vi "obstacle1.vi"(9 "Boolean":bool, 10 "f":i32, 11 "Position in":T1) -> (0 "deliver":bool, 3 "Position out":T1)   [LabVIEW 2014]
uses:
  <vilib>/Utility/miscctls.llb/LVPositionTypeDef.ctl
panel:
  out "skill":bool
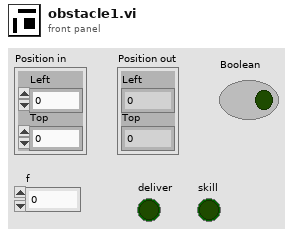
[diagram p1: front panel]
types:
  T1 = typedef "LVPositionTypeDef.ctl" = cluster{"Left":i32, "Top":i32}
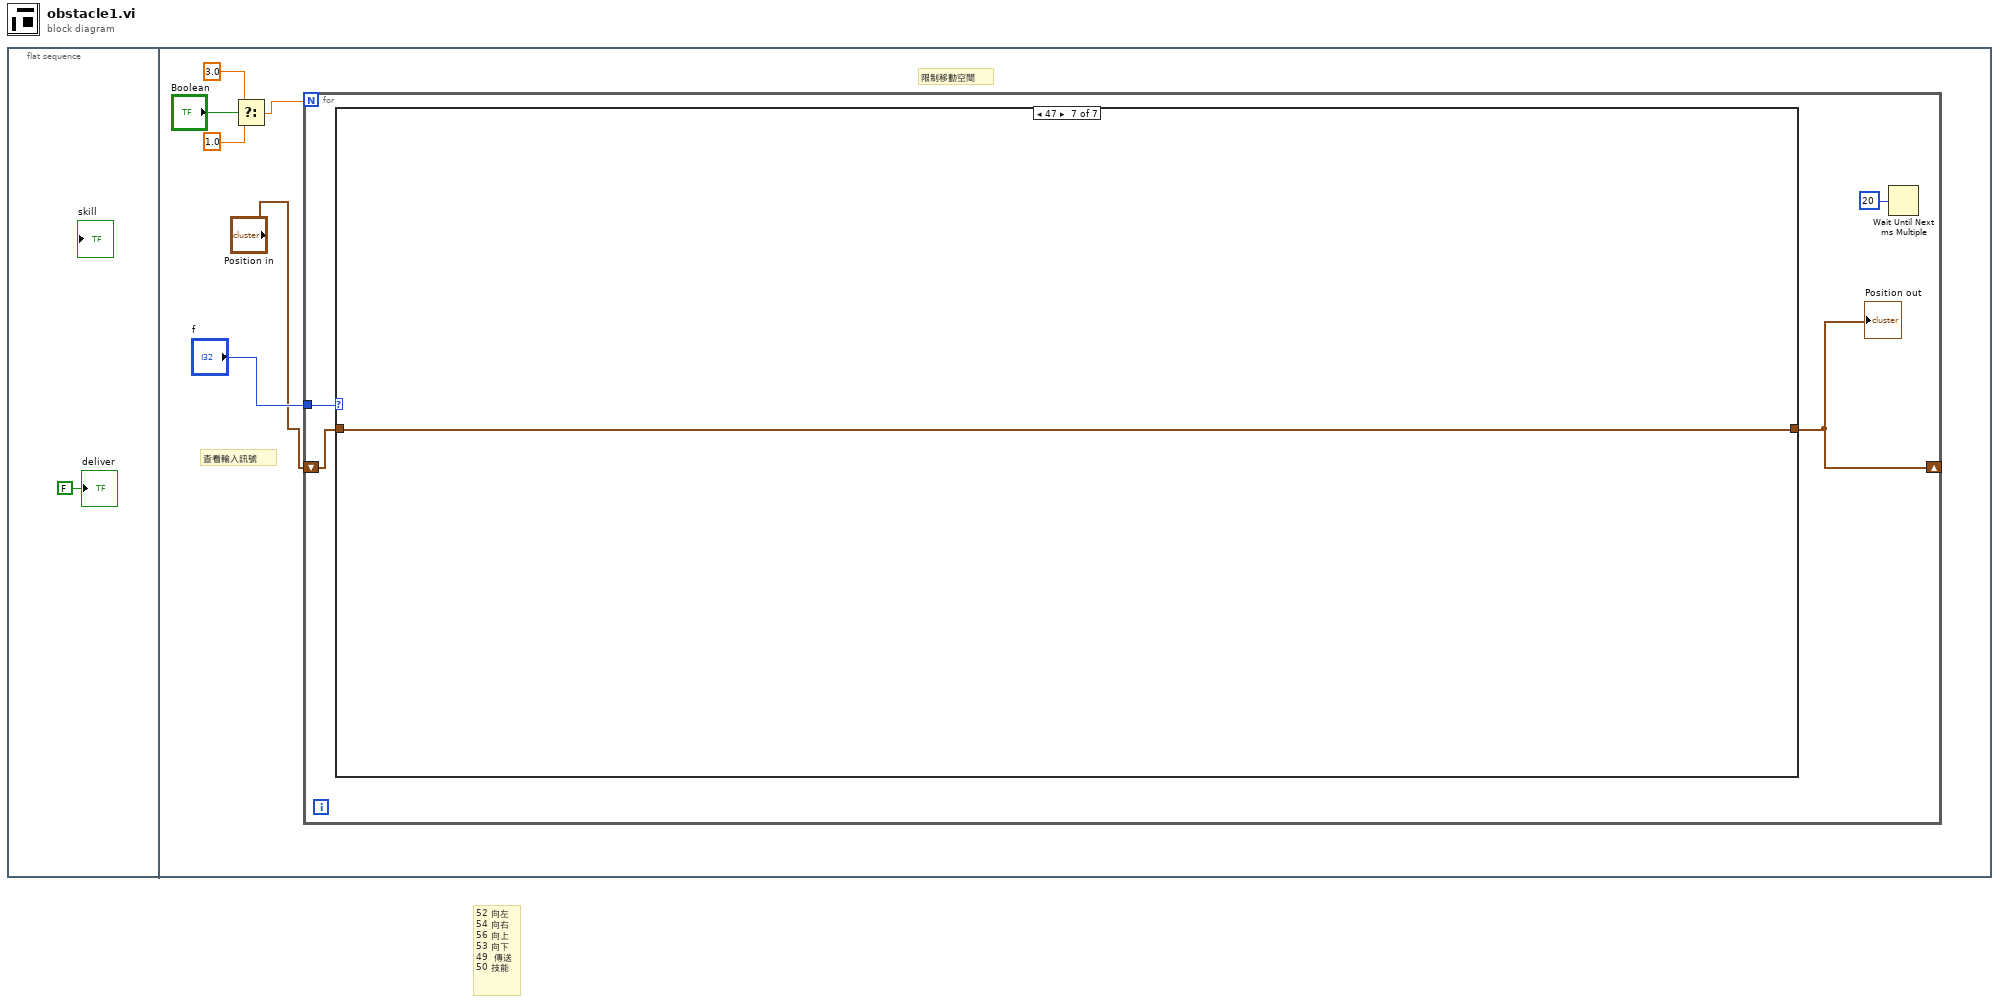
[diagram p0: block diagram]
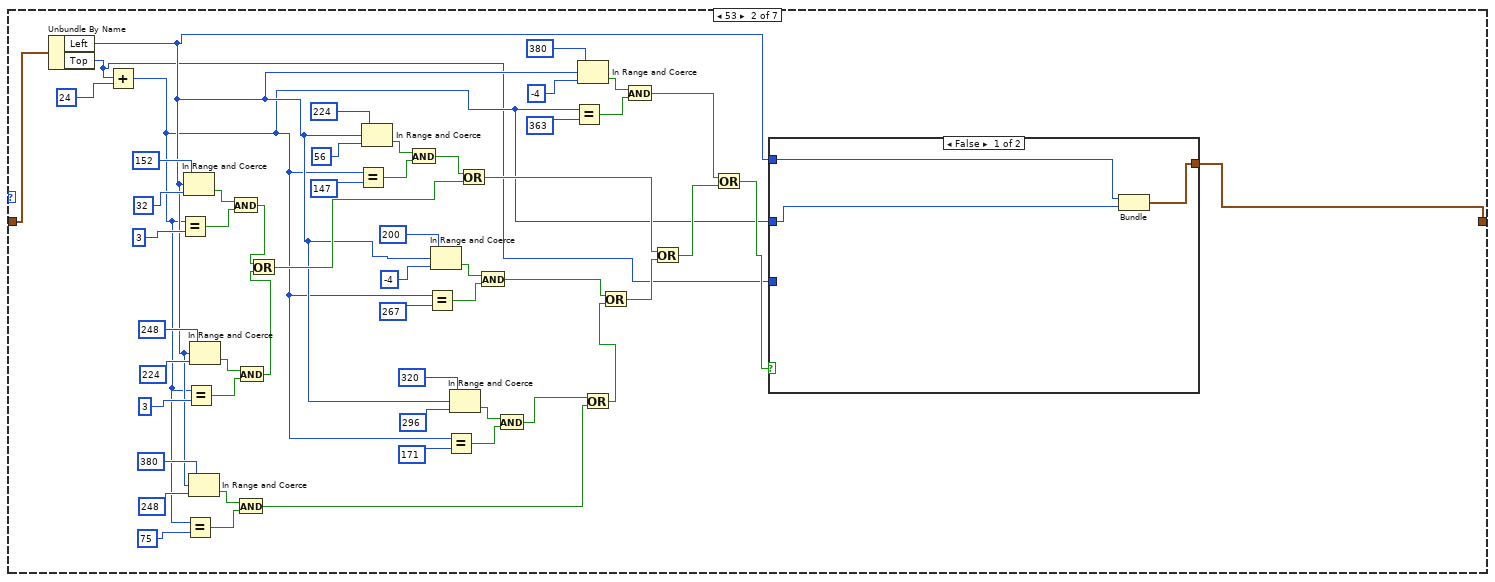
[diagram p3: hidden frame]
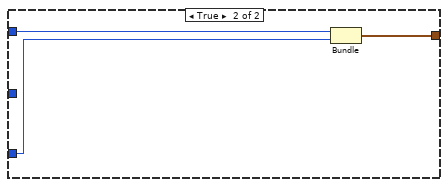
[diagram p4: hidden frame]
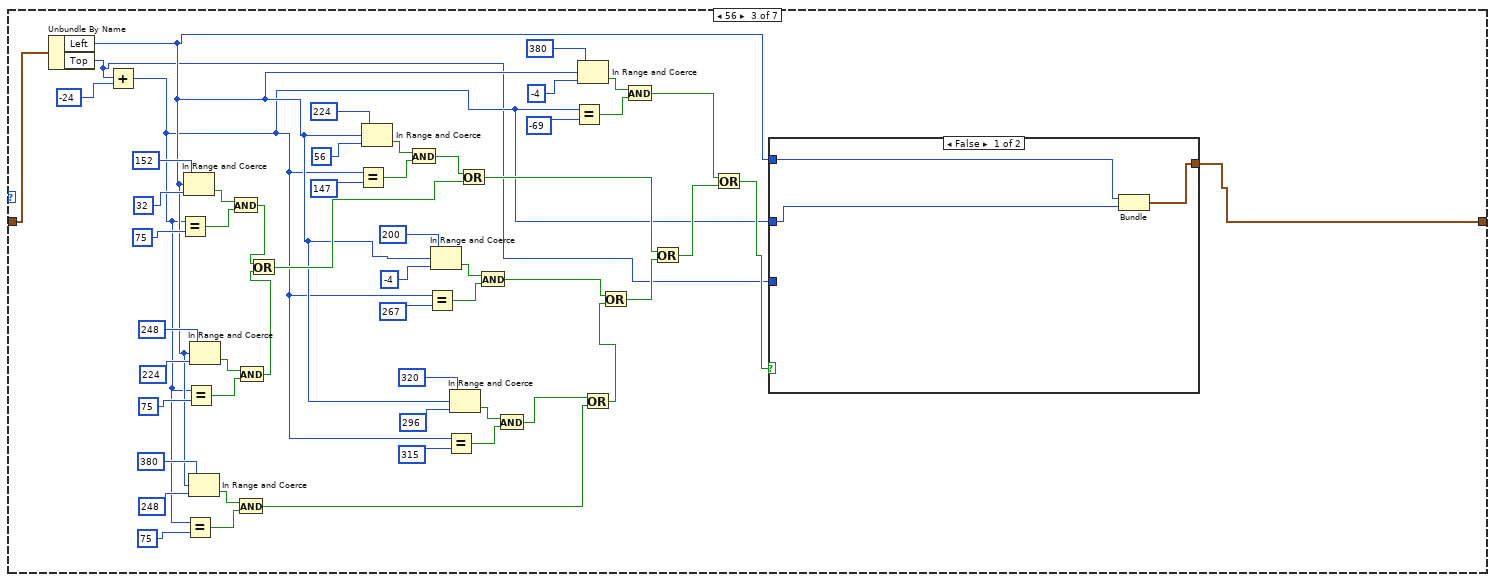
[diagram p5: hidden frame]
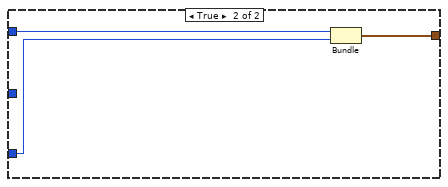
[diagram p6: hidden frame]
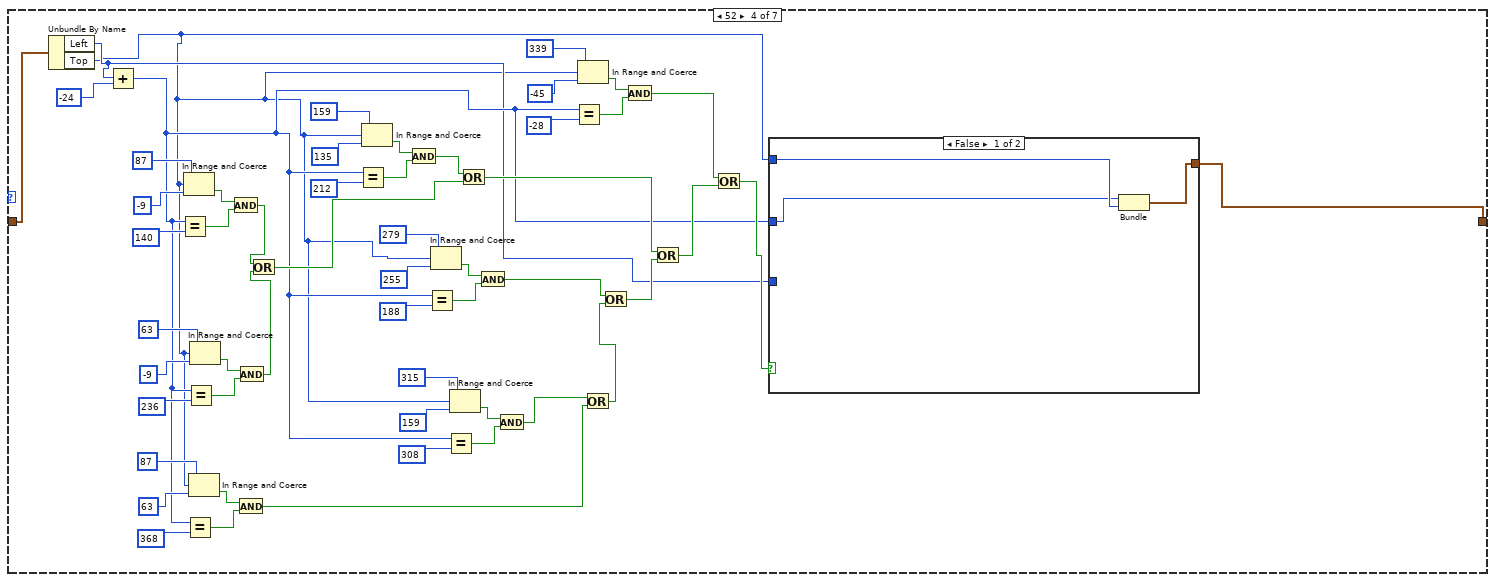
[diagram p7: hidden frame]
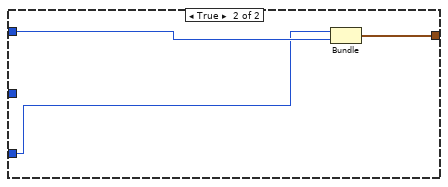
[diagram p8: hidden frame]
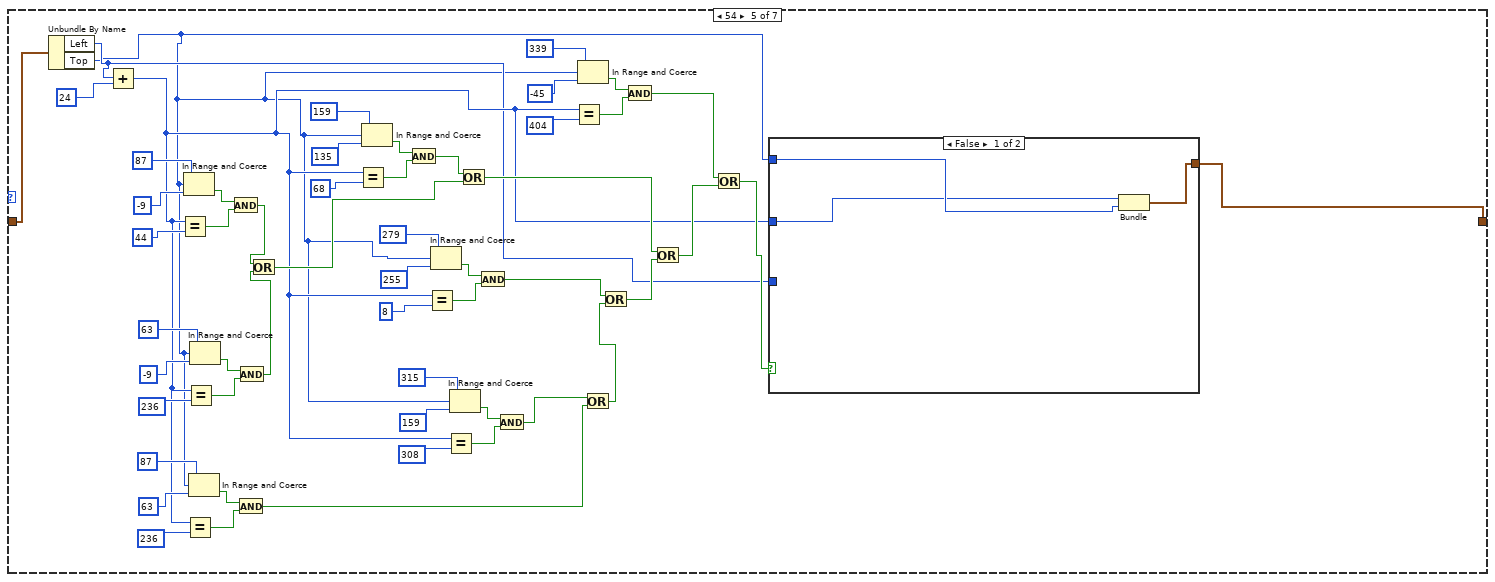
[diagram p9: hidden frame]
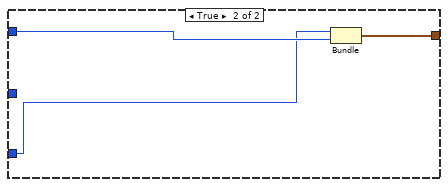
[diagram p10: hidden frame]
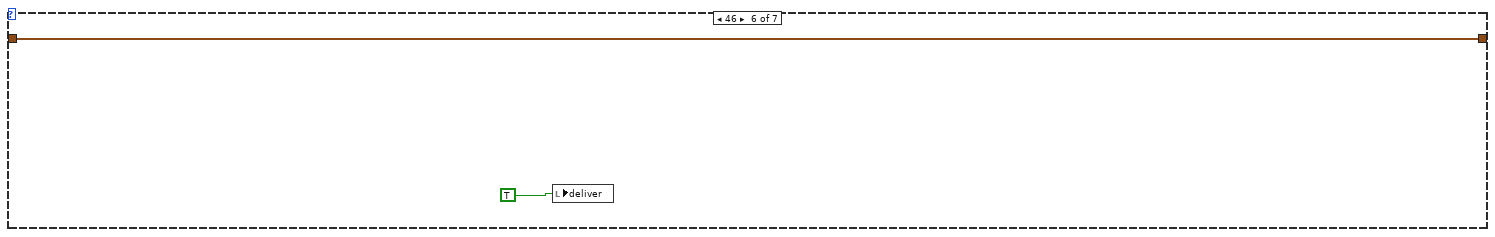
[diagram p11: hidden frame]
diagram:
  # "52 向左\n54 向右\n56 向上\n53 向下\n49  傳送\n50 技能"
  n1 = flat-sequence {
    frame #0 {
      "deliver" <- FALSE ("skill")
    }
    frame #1 {
      # "限制移動空間"
      # "查看輸入訊號"
      n2 = Select(t=3.0, s="Boolean", f=1.0) -> (s? t:f=w3:dbl)
      n3 = for {
        N: w3 -> [_]
        tunnel: "f" -> [w11]
        shift-right: [w10] -> _
        shift-left: "Position in" -> [w9]
        n4 = case shown="47" w11 {
          tunnel: w9 -> [w12 w65 w125 w185 w245 w254 w255]
          tunnel: [w12 w64 w73 w184 w244 w254 w255] -> w10
          frame 0, Default {
          }
          frame 53 {
            n5 = Unbundle By Name(w65) -> ("Left"=w15:i32, "Top"=w13:i32)
            n6 = Add(x=w13, y=24) -> (x+y=w14:i32)
            n7 = Equal?(x=w14, y=3) -> (x = y?=w60:bool)
            n8 = In Range and Coerce(upper limit=152, x=w15, lower limit=32) -> (In Range?=w59:bool)  [unwired: 1 out]
            n9 = Equal?(x=w14, y=75) -> (x = y?=w50:bool)
            n10 = Equal?(x=w14, y=3) -> (x = y?=w55:bool)
            n11 = In Range and Coerce(upper limit=380, x=w15, lower limit=248) -> (In Range?=w49:bool)  [unwired: 1 out]
            n12 = In Range and Coerce(upper limit=248, x=w15, lower limit=224) -> (In Range?=w54:bool)  [unwired: 1 out]
            n13 = And(x=w59, y=w60) -> (x .and. y?=w33:bool)
            n14 = And(x=w49, y=w50) -> (x .and. y?=w29:bool)
            n15 = And(x=w54, y=w55) -> (x .and. y?=w32:bool)
            n16 = Or(x=w33, y=w32) -> (x .or. y?=w31:bool)
            n17 = Equal?(x=w14, y=147) -> (x = y?=w45:bool)
            n18 = In Range and Coerce(upper limit=224, x=w15, lower limit=56) -> (In Range?=w44:bool)  [unwired: 1 out]
            n19 = And(x=w44, y=w45) -> (x .and. y?=w30:bool)
            n20 = Equal?(x=w14, y=267) -> (x = y?=w40:bool)
            n21 = In Range and Coerce(upper limit=200, x=w15, lower limit=-4) -> (In Range?=w39:bool)  [unwired: 1 out]
            n22 = Equal?(x=w14, y=171) -> (x = y?=w35:bool)
            n23 = In Range and Coerce(upper limit=320, x=w15, lower limit=296) -> (In Range?=w34:bool)  [unwired: 1 out]
            n24 = Or(x=w30, y=w31) -> (x .or. y?=w24:bool)
            n25 = And(x=w39, y=w40) -> (x .and. y?=w27:bool)
            n26 = And(x=w34, y=w35) -> (x .and. y?=w28:bool)
            n27 = Equal?(x=w14, y=363) -> (x = y?=w20:bool)
            n28 = In Range and Coerce(upper limit=380, x=w15, lower limit=-4) -> (In Range?=w19:bool)  [unwired: 1 out]
            n29 = Or(x=w28, y=w29) -> (x .or. y?=w26:bool)
            n30 = Or(x=w27, y=w26) -> (x .or. y?=w25:bool)
            n31 = And(x=w19, y=w20) -> (x .and. y?=w18:bool)
            n32 = Or(x=w24, y=w25) -> (x .or. y?=w17:bool)
            n33 = Or(x=w18, y=w17) -> (x .or. y?=w16:bool)
            n34 = case shown="False" w16 {
              tunnel: w15 -> [w68 w71]
              tunnel: [w69 w72] -> w64
              tunnel: w14 -> [w67 _]
              tunnel: w13 -> [_ w70]
              frame False {
                n35 = Bundle("Left"=w68, w67) -> (w69:cluster{"Left":i32, i32})  [unwired: 1 in]
              }
              frame True {
                n36 = Bundle("Left"=w71, "Top"=w70) -> (w72:cluster{"Left":i32, "Top":i32})  [unwired: 1 in]
              }
            }
          }
          frame 56 {
            n37 = Unbundle By Name(w125) -> ("Left"=w76:i32, "Top"=w74:i32)
            n38 = Add(x=w74, y=-24) -> (x+y=w75:i32)
            n39 = Equal?(x=w75, y=75) -> (x = y?=w121:bool)
            n40 = In Range and Coerce(upper limit=152, x=w76, lower limit=32) -> (In Range?=w120:bool)  [unwired: 1 out]
            n41 = Equal?(x=w75, y=75) -> (x = y?=w111:bool)
            n42 = Equal?(x=w75, y=75) -> (x = y?=w116:bool)
            n43 = In Range and Coerce(upper limit=380, x=w76, lower limit=248) -> (In Range?=w110:bool)  [unwired: 1 out]
            n44 = In Range and Coerce(upper limit=248, x=w76, lower limit=224) -> (In Range?=w115:bool)  [unwired: 1 out]
            n45 = And(x=w120, y=w121) -> (x .and. y?=w94:bool)
            n46 = And(x=w110, y=w111) -> (x .and. y?=w90:bool)
            n47 = And(x=w115, y=w116) -> (x .and. y?=w93:bool)
            n48 = Or(x=w94, y=w93) -> (x .or. y?=w92:bool)
            n49 = Equal?(x=w75, y=147) -> (x = y?=w106:bool)
            n50 = In Range and Coerce(upper limit=224, x=w76, lower limit=56) -> (In Range?=w105:bool)  [unwired: 1 out]
            n51 = And(x=w105, y=w106) -> (x .and. y?=w91:bool)
            n52 = Equal?(x=w75, y=267) -> (x = y?=w101:bool)
            n53 = In Range and Coerce(upper limit=200, x=w76, lower limit=-4) -> (In Range?=w100:bool)  [unwired: 1 out]
            n54 = Equal?(x=w75, y=315) -> (x = y?=w96:bool)
            n55 = In Range and Coerce(upper limit=320, x=w76, lower limit=296) -> (In Range?=w95:bool)  [unwired: 1 out]
            n56 = Or(x=w91, y=w92) -> (x .or. y?=w85:bool)
            n57 = And(x=w100, y=w101) -> (x .and. y?=w88:bool)
            n58 = And(x=w95, y=w96) -> (x .and. y?=w89:bool)
            n59 = Equal?(x=w75, y=-69) -> (x = y?=w81:bool)
            n60 = In Range and Coerce(upper limit=380, x=w76, lower limit=-4) -> (In Range?=w80:bool)  [unwired: 1 out]
            n61 = Or(x=w89, y=w90) -> (x .or. y?=w87:bool)
            n62 = Or(x=w88, y=w87) -> (x .or. y?=w86:bool)
            n63 = And(x=w80, y=w81) -> (x .and. y?=w79:bool)
            n64 = Or(x=w85, y=w86) -> (x .or. y?=w78:bool)
            n65 = Or(x=w79, y=w78) -> (x .or. y?=w77:bool)
            n66 = case shown="False" w77 {
              tunnel: w76 -> [w128 w131]
              tunnel: [w129 w132] -> w73
              tunnel: w75 -> [w127 _]
              tunnel: w74 -> [_ w130]
              frame False {
                n67 = Bundle("Left"=w128, w127) -> (w129:cluster{"Left":i32, i32})  [unwired: 1 in]
              }
              frame True {
                n68 = Bundle("Left"=w131, "Top"=w130) -> (w132:cluster{"Left":i32, "Top":i32})  [unwired: 1 in]
              }
            }
          }
          frame 52 {
            n69 = Unbundle By Name(w185) -> ("Left"=w134:i32, "Top"=w133:i32)
            n70 = Add(x=w134, y=-24) -> (x+y=w135:i32)
            n71 = Equal?(x=w135, y=140) -> (x = y?=w180:bool)
            n72 = In Range and Coerce(upper limit=87, x=w133, lower limit=-9) -> (In Range?=w179:bool)  [unwired: 1 out]
            n73 = Equal?(x=w135, y=368) -> (x = y?=w170:bool)
            n74 = Equal?(x=w135, y=236) -> (x = y?=w175:bool)
            n75 = In Range and Coerce(upper limit=87, x=w133, lower limit=63) -> (In Range?=w169:bool)  [unwired: 1 out]
            n76 = In Range and Coerce(upper limit=63, x=w133, lower limit=-9) -> (In Range?=w174:bool)  [unwired: 1 out]
            n77 = And(x=w179, y=w180) -> (x .and. y?=w153:bool)
            n78 = And(x=w169, y=w170) -> (x .and. y?=w149:bool)
            n79 = And(x=w174, y=w175) -> (x .and. y?=w152:bool)
            n80 = Or(x=w153, y=w152) -> (x .or. y?=w151:bool)
            n81 = Equal?(x=w135, y=212) -> (x = y?=w165:bool)
            n82 = In Range and Coerce(upper limit=159, x=w133, lower limit=135) -> (In Range?=w164:bool)  [unwired: 1 out]
            n83 = And(x=w164, y=w165) -> (x .and. y?=w150:bool)
            n84 = Equal?(x=w135, y=188) -> (x = y?=w160:bool)
            n85 = In Range and Coerce(upper limit=279, x=w133, lower limit=255) -> (In Range?=w159:bool)  [unwired: 1 out]
            n86 = Equal?(x=w135, y=308) -> (x = y?=w155:bool)
            n87 = In Range and Coerce(upper limit=315, x=w133, lower limit=159) -> (In Range?=w154:bool)  [unwired: 1 out]
            n88 = Or(x=w150, y=w151) -> (x .or. y?=w144:bool)
            n89 = And(x=w159, y=w160) -> (x .and. y?=w147:bool)
            n90 = And(x=w154, y=w155) -> (x .and. y?=w148:bool)
            n91 = Equal?(x=w135, y=-28) -> (x = y?=w140:bool)
            n92 = In Range and Coerce(upper limit=339, x=w133, lower limit=-45) -> (In Range?=w139:bool)  [unwired: 1 out]
            n93 = Or(x=w148, y=w149) -> (x .or. y?=w146:bool)
            n94 = Or(x=w147, y=w146) -> (x .or. y?=w145:bool)
            n95 = And(x=w139, y=w140) -> (x .and. y?=w138:bool)
            n96 = Or(x=w144, y=w145) -> (x .or. y?=w137:bool)
            n97 = Or(x=w138, y=w137) -> (x .or. y?=w136:bool)
            n98 = case shown="False" w136 {
              tunnel: w133 -> [w188 w191]
              tunnel: [w189 w192] -> w184
              tunnel: w135 -> [w187 _]
              tunnel: w134 -> [_ w190]
              frame False {
                n99 = Bundle(w187, "Top"=w188) -> (w189:cluster{i32, "Top":i32})  [unwired: 1 in]
              }
              frame True {
                n100 = Bundle("Left"=w190, "Top"=w191) -> (w192:cluster{"Left":i32, "Top":i32})  [unwired: 1 in]
              }
            }
          }
          frame 54 {
            n101 = Unbundle By Name(w245) -> ("Left"=w194:i32, "Top"=w193:i32)
            n102 = Add(x=w194, y=24) -> (x+y=w195:i32)
            n103 = Equal?(x=w195, y=44) -> (x = y?=w240:bool)
            n104 = In Range and Coerce(upper limit=87, x=w193, lower limit=-9) -> (In Range?=w239:bool)  [unwired: 1 out]
            n105 = Equal?(x=w195, y=236) -> (x = y?=w230:bool)
            n106 = Equal?(x=w195, y=236) -> (x = y?=w235:bool)
            n107 = In Range and Coerce(upper limit=87, x=w193, lower limit=63) -> (In Range?=w229:bool)  [unwired: 1 out]
            n108 = In Range and Coerce(upper limit=63, x=w193, lower limit=-9) -> (In Range?=w234:bool)  [unwired: 1 out]
            n109 = And(x=w239, y=w240) -> (x .and. y?=w213:bool)
            n110 = And(x=w229, y=w230) -> (x .and. y?=w209:bool)
            n111 = And(x=w234, y=w235) -> (x .and. y?=w212:bool)
            n112 = Or(x=w213, y=w212) -> (x .or. y?=w211:bool)
            n113 = Equal?(x=w195, y=68) -> (x = y?=w225:bool)
            n114 = In Range and Coerce(upper limit=159, x=w193, lower limit=135) -> (In Range?=w224:bool)  [unwired: 1 out]
            n115 = And(x=w224, y=w225) -> (x .and. y?=w210:bool)
            n116 = Equal?(x=w195, y=8) -> (x = y?=w220:bool)
            n117 = In Range and Coerce(upper limit=279, x=w193, lower limit=255) -> (In Range?=w219:bool)  [unwired: 1 out]
            n118 = Equal?(x=w195, y=308) -> (x = y?=w215:bool)
            n119 = In Range and Coerce(upper limit=315, x=w193, lower limit=159) -> (In Range?=w214:bool)  [unwired: 1 out]
            n120 = Or(x=w210, y=w211) -> (x .or. y?=w204:bool)
            n121 = And(x=w219, y=w220) -> (x .and. y?=w207:bool)
            n122 = And(x=w214, y=w215) -> (x .and. y?=w208:bool)
            n123 = Equal?(x=w195, y=404) -> (x = y?=w200:bool)
            n124 = In Range and Coerce(upper limit=339, x=w193, lower limit=-45) -> (In Range?=w199:bool)  [unwired: 1 out]
            n125 = Or(x=w208, y=w209) -> (x .or. y?=w206:bool)
            n126 = Or(x=w207, y=w206) -> (x .or. y?=w205:bool)
            n127 = And(x=w199, y=w200) -> (x .and. y?=w198:bool)
            n128 = Or(x=w204, y=w205) -> (x .or. y?=w197:bool)
            n129 = Or(x=w198, y=w197) -> (x .or. y?=w196:bool)
            n130 = case shown="False" w196 {
              tunnel: w193 -> [w248 w251]
              tunnel: [w249 w252] -> w244
              tunnel: w195 -> [w247 _]
              tunnel: w194 -> [_ w250]
              frame False {
                n131 = Bundle(w247, "Top"=w248) -> (w249:cluster{i32, "Top":i32})  [unwired: 1 in]
              }
              frame True {
                n132 = Bundle("Left"=w250, "Top"=w251) -> (w252:cluster{"Left":i32, "Top":i32})  [unwired: 1 in]
              }
            }
          }
          frame 46 {
            n133 = local write "deliver"(TRUE ("skill")) -> ()
          }
          frame 47 {
          }
        }
        "Position out" <- w10
        n134 = Wait Until Next ms Multiple(millisecond multiple=u32 20) -> ()  [unwired: 1 out]
      }
    }
  }
